vi "send_translation_request.vi"(8 "error in (no error)":errorcluster, 9 "translation mode":T1, 10 "translation vector":refnum<class "SpaceVector.lvclass">, 11 "GenericStage in":refnum<class "GenericStage.lvclass">) -> (0 "error out":errorcluster, 3 "GenericStage out":refnum<class "GenericStage.lvclass">)   [LabVIEW 2010, in "GenericStage.lvclass"]
uses:
  GenericStage.lvclass
  common/classes/SpaceVector/SpaceVector/SpaceVector.lvclass
  translation_mode_enum.ctl
  trigger_enum.ctl
  translation_request.ctl
  class_data.vi
  common/classes/ErrorController/ErrorController/class_data.vi
  common/classes/ErrorController/ErrorController/ErrorController.lvclass
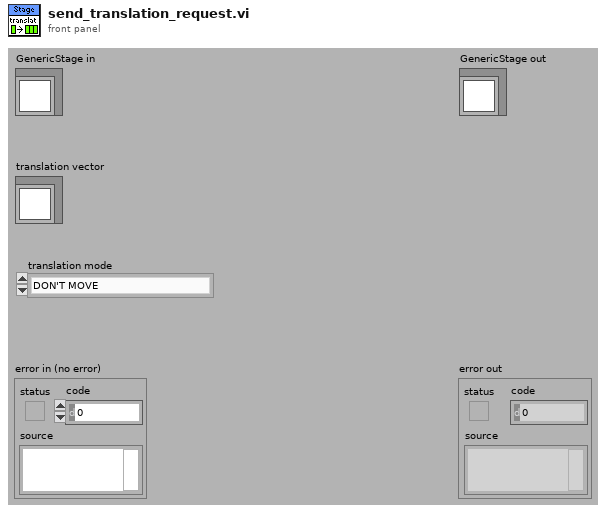
[diagram p1: front panel]
types:
  T1 = typedef "GenericStage.lvclass/translation_mode_enum.ctl" = enum16{"DON'T MOVE", "relative", "absolute"}
  T2 = typedef "GenericStage.lvclass/trigger_enum.ctl" = enum16{"NULL", "move", "update position", "set origin", "return to origin"}
  T3 = typedef "GenericStage.lvclass/translation_request.ctl" = cluster{"translation mode":T1, "translation vector":refnum<class "SpaceVector.lvclass">}
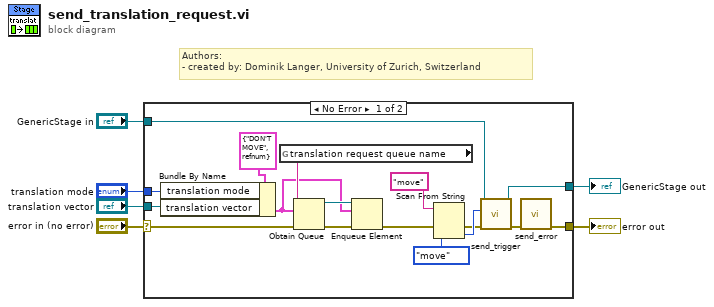
[diagram p0: block diagram]
diagram:
  # "Authors: \n- created by: Dominik Langer, University of Zurich, Switzerland"
  n1 = case shown="No Error" "error in (no error)" {
    selector: "error in (no error)" -> [w17 w25]
    tunnel: [w12 w25] -> w5
    tunnel: [w14 w24] -> w3
    tunnel: "GenericStage in" -> [w15 w24]
    tunnel: "translation mode" -> [w22 _]
    tunnel: "translation vector" -> [w21 _]
    frame No Error {
      n2 = Bundle By Name(cluster=T3 {"translation mode"=enum."DON'T MOVE", "translation vector"=refnum} ("translation request"), "translation mode"=w22, "translation vector"=w21) -> (w16:T3)
      n3 = global read "class_data.vi" "translation request queue name"() -> (w20:string)
      n4 = Obtain Queue(name (unnamed)=w20, element data type=w16, error in (no error)=w17) -> (queue out=w19:refnum<queue>, error out=w18:errorcluster)  [unwired: 2 in, 1 out]
      n5 = Enqueue Element(queue=w19, element=w16, error in (no error)=w18) -> (error out=w8:errorcluster)  [unwired: 1 in, 2 out]
      n6 = Scan From String(input string="move", error in=w8, default 1=trigger_enum."move" ("trigger")) -> (error out=w9:errorcluster, output 1=w11:T2)  [unwired: 2 in, 2 out]
      n7 = call-dynamic "send_trigger.vi"("error in (no error)"=w9, "trigger"=w11, "GenericStage in"=w15) -> ("error out"=w13:errorcluster, "GenericStage out"=w14:refnum<class "GenericStage.lvclass">)  [unwired: 7 out]
      n8 = call "send_error.vi"("error in (no error)"=w13) -> ("error out"=w12:errorcluster)  [unwired: 10 in]
    }
    frame Error {
    }
  }
  "error out" <- w5
  "GenericStage out" <- w3
